vi "TestRFGVRequests.vi"() -> ()   [LabVIEW 2015]
uses:
  TypeDef/RoomsActionEnum.ctl
  LVClasses/Request/PersonnelType.ctl
  LVClasses/Request/RequestType.ctl
  LVClasses/Request/Request.lvclass/Request.ctl
  LVClasses/Request/Read Summary.vi
  LVClasses/Request/Request.lvclass
panel:
  out "Remove":bool
  out "Add":bool
  out "Add Request 2":string
  out "Read Request 3":string
  out "Remove Request":string
  out "Add Request 1":string
  out "Read Requests 1":string
  out "Read Requests 2":string
  out "error out":errorcluster
  out "Pass":bool
  in  "Rooms":i32=101
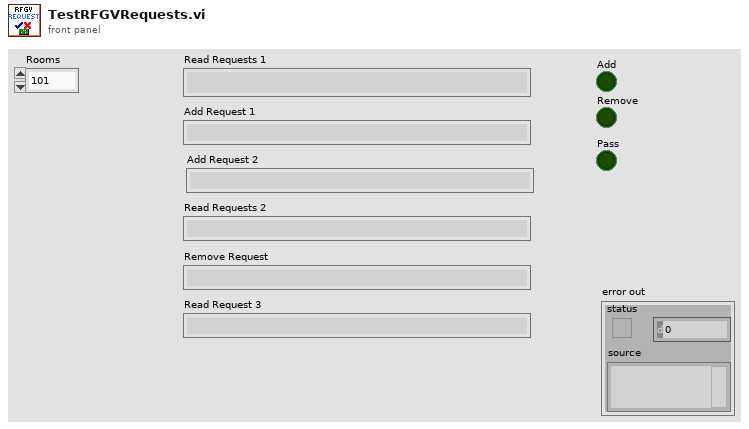
[diagram p1: front panel]
types:
  T1 = typedef "Request.lvclass/RequestType.ctl" = enum16{"Specific Call To Room", "General Call To Room"}
  T2 = typedef "Request.lvclass/PersonnelType.ctl" = u16
  T3 = typedef "RoomsActionEnum.ctl" = enum16{"Init", "Add Room", "Remove Room", "Read Room", "Read Flag", "Read Flag State", "Write Flag State", "Read Flag Color", "Write Flag Color", "Read Bed Vacant", "Write Bed Vacant", "Read Personnel", "Add Personnel", "Remove Personnel", "Read Requests", "Add Request", "Remove Request", "Read Beacon ID", "Write Beacon ID", "Write Bed URL", "Read Bed URL", "Read Rooms Numbers", "Write Flag"}
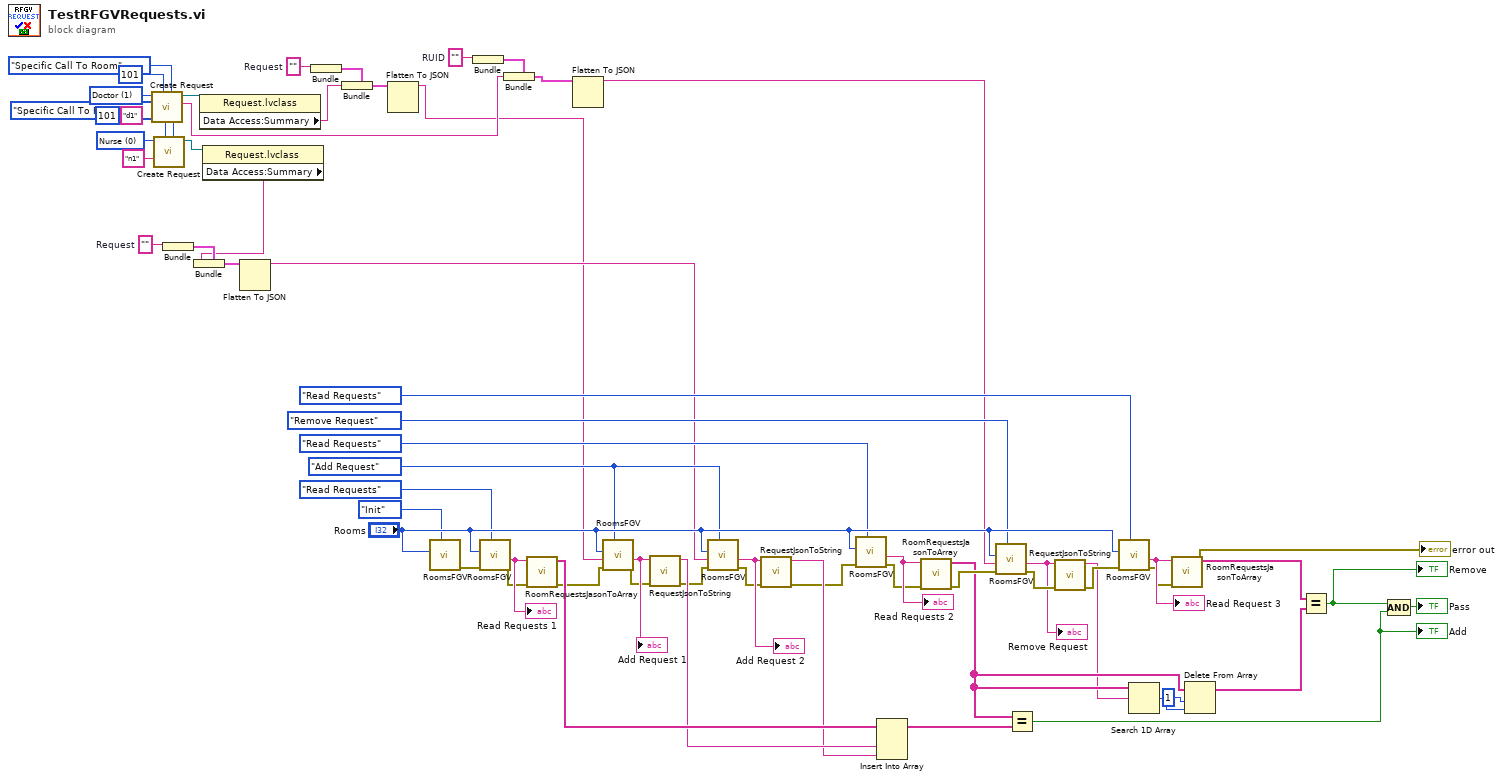
[diagram p0: block diagram]
diagram:
  w7 = ""  # RUID
  w16 = T2 0 items=["Nurse", "Doctor", "Cleanning", "Admin"] ("Personnel Type")
  w17 = T2 1 items=["Nurse", "Doctor", "Cleanning", "Admin"] ("Personnel Type")
  w20 = ""  # Request
  w25 = ""  # Request
  w29 = RoomsActionEnum."Add Request" ("Actions")
  n1 = call "Create Request.vi"("Request Type"=RequestType."Specific Call To Room", "Room Number"=101, "Name"="d1", "Personnel Type"=w17) -> ("RUID"=w5:string, "Request out"=w18:refnum<class "Request.lvclass">)  [unwired: 5 in, 1 out]
  n2 = call "Create Request.vi"("Request Type"=RequestType."Specific Call To Room", "Room Number"=101, "Name"="n1", "Personnel Type"=w16) -> ("Request out"=w19:refnum<class "Request.lvclass">)  [unwired: 5 in, 2 out]
  n3 = Bundle("Request"=w20) -> (w21:cluster{"Request":string})  [unwired: 1 in]
  n4 = property class="Request.lvclass"(reference=w18) -> ("Data Access:Summary"=w9:string)  [unwired: 1 in, 2 out]
  n5 = property class="Request.lvclass"(reference=w19) -> ("Data Access:Summary"=w8:string)  [unwired: 1 in, 2 out]
  n6 = Bundle(cluster=w21, "Request"=w8) -> (w22:cluster{"Request":string})
  n7 = Flatten To JSON(anything=w22) -> (JSON string=w3:string)  [unwired: 2 in, 1 out]
  n8 = Bundle("Request"=w25) -> (w24:cluster{"Request":string})  [unwired: 1 in]
  n9 = Bundle(cluster=w24, "Request"=w9) -> (w23:cluster{"Request":string})
  n10 = Flatten To JSON(anything=w23) -> (JSON string=w2:string)  [unwired: 2 in, 1 out]
  n11 = call "RoomsFGV.vi"("Actions"=RoomsActionEnum."Init", "Room"="Rooms") -> ("error out"=w64:errorcluster)  [unwired: 8 in, 1 out]
  n12 = Bundle("RUID"=w7) -> (w6:cluster{"RUID":string})  [unwired: 1 in]
  n13 = call "RoomsFGV.vi"("Actions"=RoomsActionEnum."Read Requests", "error in (no error)"=w64, "Room"="Rooms") -> ("error out"=w53:errorcluster, "Data Out"=w59:string)  [unwired: 7 in]
  "Read Requests 1" <- w59
  n14 = Bundle(cluster=w6, "RUID"=w5) -> (w4:cluster{"RUID":string})
  n15 = call "RoomRequestsJasonToArray.vi"("error in (no error)"=w53, "Data Out"=w59) -> ("error out"=w52:errorcluster, "REQs"=w58:string[])  [unwired: 8 in]
  n16 = Flatten To JSON(anything=w4) -> (JSON string=w1:string)  [unwired: 2 in, 1 out]
  n17 = call "RoomsFGV.vi"("Actions"=w29, "error in (no error)"=w52, "Data In"=w2, "Room"="Rooms") -> ("error out"=w51:errorcluster, "Data Out"=w61:string)  [unwired: 6 in]
  "Add Request 1" <- w61
  n18 = call "RequestJsonToString.vi"("error in (no error)"=w51, "Data Out"=w61) -> ("error out"=w50:errorcluster, "Request"=w57:string)  [unwired: 8 in]
  n19 = call "RoomsFGV.vi"("Actions"=w29, "error in (no error)"=w50, "Data In"=w3, "Room"="Rooms") -> ("error out"=w49:errorcluster, "Data Out"=w60:string)  [unwired: 6 in]
  "Add Request 2" <- w60
  n20 = call "RequestJsonToString.vi"("error in (no error)"=w49, "Data Out"=w60) -> ("error out"=w48:errorcluster, "Request"=w56:string)  [unwired: 8 in]
  n21 = call "RoomsFGV.vi"("Actions"=RoomsActionEnum."Read Requests", "error in (no error)"=w48, "Room"="Rooms") -> ("error out"=w47:errorcluster, "Data Out"=w55:string)  [unwired: 7 in]
  "Read Requests 2" <- w55
  n22 = Insert Into Array(array=w58, new element #1=w57, new element #2=w56) -> (w54:string[])  [unwired: 1 in]
  n23 = call "RoomRequestsJasonToArray.vi"("error in (no error)"=w47, "Data Out"=w55) -> ("error out"=w46:errorcluster, "REQs"=w40:string[])  [unwired: 8 in]
  n24 = call "RoomsFGV.vi"("Actions"=RoomsActionEnum."Remove Request", "error in (no error)"=w46, "Data In"=w1, "Room"="Rooms") -> ("error out"=w45:errorcluster, "Data Out"=w43:string)  [unwired: 6 in]
  "Remove Request" <- w43
  n25 = Equal?(x=w40, y=w54) -> (x = y?=w62:bool)
  "Add" <- w62
  n26 = call "RequestJsonToString.vi"("error in (no error)"=w45, "Data Out"=w43) -> ("error out"=w44:errorcluster, "Request"=w39:string)  [unwired: 8 in]
  n27 = call "RoomsFGV.vi"("Actions"=RoomsActionEnum."Read Requests", "error in (no error)"=w44, "Room"="Rooms") -> ("error out"=w37:errorcluster, "Data Out"=w38:string)  [unwired: 7 in]
  "Read Request 3" <- w38
  n28 = Search 1D Array(1D array=w40, element=w39) -> (index of element=w42:i32)  [unwired: 1 in]
  n29 = call "RoomRequestsJasonToArray.vi"("error in (no error)"=w37, "Data Out"=w38) -> ("error out"=→"error out":errorcluster, "REQs"=w35:string[])  [unwired: 8 in]
  n30 = Delete From Array(array=w40, length=1, index=w42) -> (array with subset deleted=w34:string[])  [unwired: 1 out]
  n31 = Equal?(x=w35, y=w34) -> (x = y?=w63:bool)
  "Remove" <- w63
  n32 = Compound Arithmetic op=AND(w63, w62) -> (→"Pass":bool)
